vi "Print Interactions.vi"(8 "error in (no error)":errorcluster, 9 "Ranges":cluster{"Upper":dbl, "Lower":dbl}[](array[cluster]), 10 "Interaction Types":string[](array[string]), 11 "Abstract Topas in":refnum<class "Abstract Topas.lvclass">) -> (0 "error out":errorcluster, 1 "Interactions Print":string, 3 "Abstract Topas out":refnum<class "Abstract Topas.lvclass">)   [LabVIEW 2020, in "Abstract Topas.lvclass"]
uses:
  Abstract Topas.lvclass
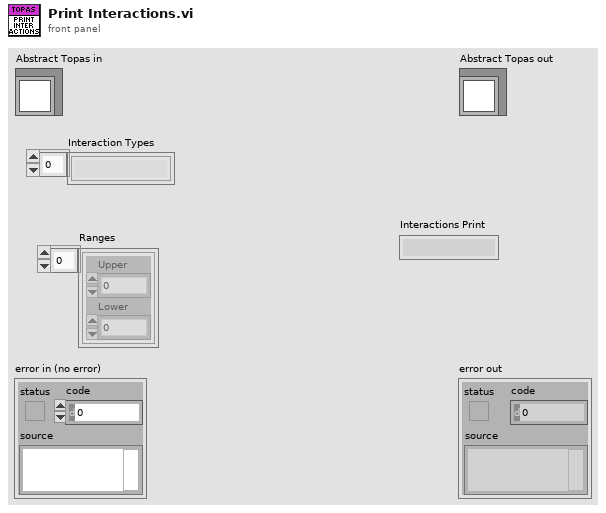
[diagram p1: front panel]
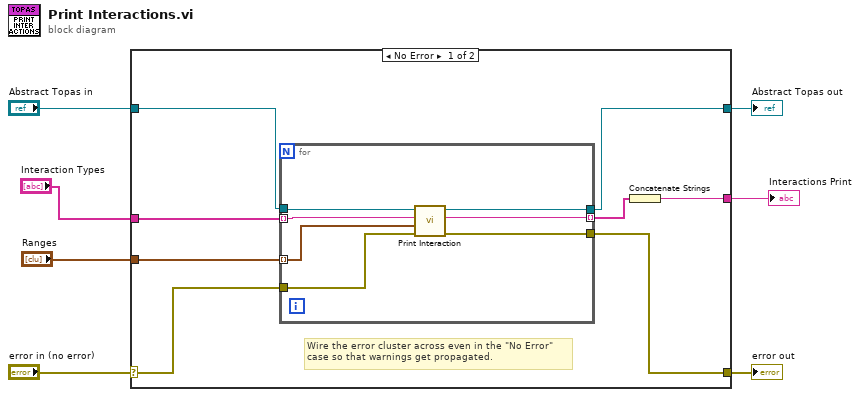
[diagram p0: block diagram]
diagram:
  n1 = case shown="No Error" "error in (no error)" {
    selector: "error in (no error)" -> [w9 w24]
    tunnel: [w8 w24] -> w6
    tunnel: [w15 w23] -> w4
    tunnel: "Abstract Topas in" -> [w14 w23]
    tunnel: "Interaction Types" -> [w13 _]
    tunnel: "Ranges" -> [w12 _]
    tunnel: [w10 _] -> w1
    frame No Error {
      # "Wire the error cluster across even in the \"No Error\"\ncase so that warnings get propagated."
      n2 = for {
        tunnel: w14 -> [w22]
        tunnel: [w21] -> w15
        tunnel: w13 -> [w20] mode=indexing
        tunnel: w12 -> [w19] mode=indexing
        tunnel: [w18] -> w11 mode=indexing
        tunnel: w9 -> [w17]
        tunnel: [w16] -> w8
        n3 = call-dynamic "Print Interaction.vi"("error in (no error)"=w17, "Range"=w19, "Interaction Type"=w20, "Abstract Topas in"=w22) -> ("error out"=w16:errorcluster, "Interaction Print"=w18:string, "Abstract Topas out"=w21:refnum<class "Abstract Topas.lvclass">)  [unwired: 5 in]
      }
      n4 = Concatenate Strings(w11) -> (w10:string)
    }
    frame Error {
    }
  }
  "error out" <- w6
  "Abstract Topas out" <- w4
  "Interactions Print" <- w1
